vi "reference_is_valid.vi"(11 "toml in":refnum<class "toml.lvclass">) -> (2 "valid refnum?":bool)   [LabVIEW 2020, in "toml.lvclass"]
uses:
  toml.lvclass
  toml.lvclass/toml.ctl
  Doc/Doc.lvclass
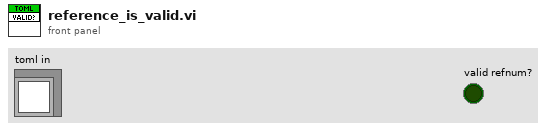
[diagram p1: front panel]
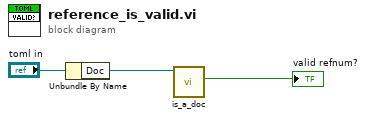
[diagram p0: block diagram]
diagram:
  n1 = Unbundle By Name("toml in") -> ("Doc"=w2:refnum<class "Doc.lvclass">)
  n2 = call "is_a_doc.vi"("Doc in"=w2) -> ("is-valid?"=→"valid refnum?":bool)  [unwired: 10 in]
